vi "Stream Arc (Polymorphic).vi"   [LabVIEW 2015, in "Zaber A Series.lvlib"]
doc: "Adds a circular arc command to an open stream. The position where the previous stream command leaves the device will be the starting point for the arc. The Center Position input specifies where the center of the circle will be, and the End Point input specified the end of the arc. There is also a Direction input to control which way around the circle the arc is drawn.\n\nThe Position Mode input controls whether the center and endpoint positions are absolute or relative to the arc start.\n\nThe center and end points are specified in microstep units - use the Convert Position to Device Units VI to convert from standard measurements.\n\nThis VI does not check in advance for error conditions such as streams not being supported or the stream not being open.\n\nThis VI requires that the Initialize VI has been called with the same serial port and that the specified stream is open."
uses:
  Zaber A Series.lvlib
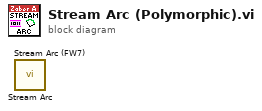
[diagram p0: block diagram]
diagram:
  n1 = call "Stream Arc.vi"() -> ()  [unwired: 10 in, 2 out]
  n2 = call "Stream Arc (FW7).vi"() -> ()  [unwired: 10 in, 2 out]
